vi "note1.vi"() -> ()   [LabVIEW 2016]
panel:
  out "Plot: All":cluster{dbl[], dbl[]}(graph)
  in  "N":i32=-1
  in  "omega0":dbl
  in  "gamma":dbl
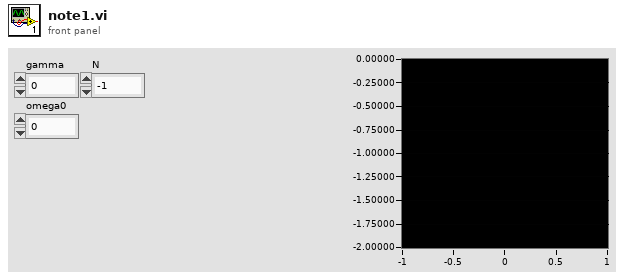
[diagram p1: front panel]
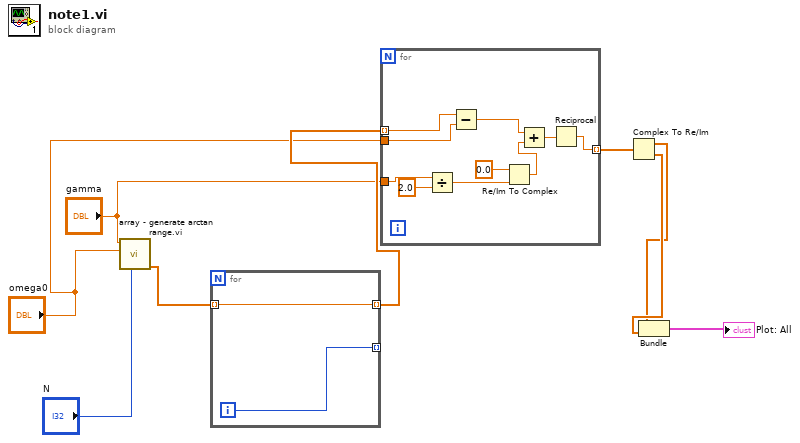
[diagram p0: block diagram]
diagram:
  n1 = call "array - generate arctan range.vi.vi"("N"="N", "omega0"="omega0", "gamma"="gamma") -> ("Array"=w8:dbl[])  [unwired: 8 in]
  n2 = for {
    tunnel: w8 -> [w10] mode=indexing
    tunnel: [w11] -> _ mode=indexing
    tunnel: [w10] -> w7 mode=indexing
    i -> [w11]
  }
  n3 = for {
    tunnel: w7 -> [w20] mode=indexing
    tunnel: "omega0" -> [w21]
    tunnel: "gamma" -> [w19]
    tunnel: [w12] -> w4 mode=indexing
    n4 = Divide(x=w19, y=2.0) -> (x/y=w17:dbl)
    n5 = Subtract(x=w20, y=w21) -> (x-y=w14:dbl)
    n6 = Re/Im To Complex(1:w17, 2:0.0 ("x")) -> (0:w15:cdb)
    n7 = Add(x=w14, y=w15) -> (x+y=w13:cdb)
    n8 = Reciprocal(x=w13) -> (1/x=w12:cdb)
  }
  n9 = Complex To Re/Im(x + iy=w4) -> (x=w2:dbl[], y=w3:dbl[])
  n10 = Bundle(w2, w3) -> (→"Plot: All":cluster{dbl[], dbl[]})  [unwired: 1 in]
